vi "Date Start (XXXXXX).vi"(10 "13:00:00":string="00:00:00", 11 "Datetime":timestamp) -> (1 "檔名":string, 3 "Date + 00:00:00":timestamp)   [LabVIEW 2019]
panel:
  out "date string":string
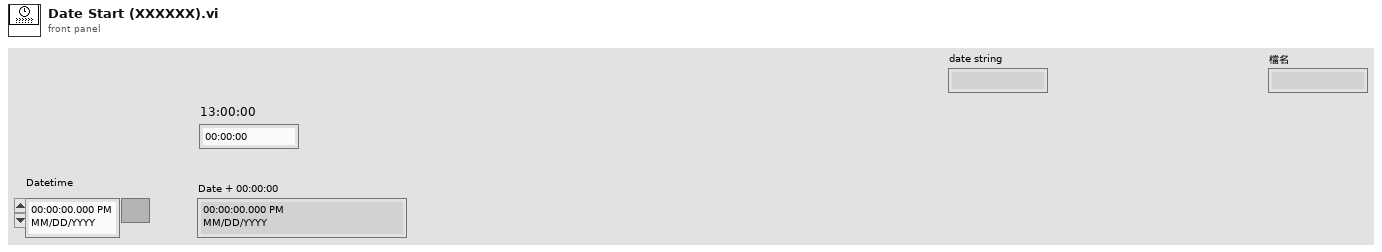
[diagram p1: front panel]
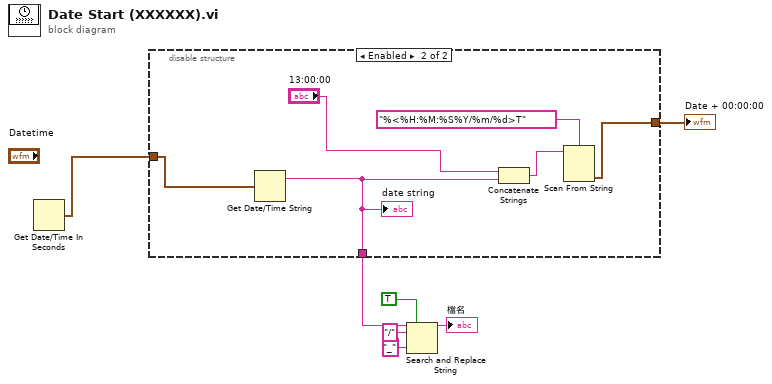
[diagram p0: block diagram]
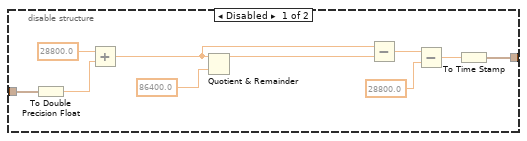
[diagram p2: hidden frame]
diagram:
  n1 = Get Date/Time In Seconds() -> (seconds since 1Jan1904=w1:timestamp)
  n2 = disable-structure shown="Enabled" {
    disable-tunnel: [w17 w20] -> w7
    disable-tunnel: w1 -> [w8 w21]
    disable-tunnel: [_ w19] -> w6
    frame Disabled {
      n3 = To Double Precision Float(number=w8) -> (double precision float=w11:dbl)
      n4 = Add(x=28800.0, y=w11) -> (x+y=w10:dbl)
      n5 = Quotient & Remainder(x=w10, y=86400.0) -> (x-y*floor(x/y)=w9:dbl)  [unwired: 1 out]
      n6 = Subtract(x=w10, y=w9) -> (x-y=w13:dbl)
      n7 = Subtract(x=w13, y=28800.0) -> (x-y=w14:dbl)
      n8 = To Time Stamp(1:w14) -> (0:w17:timestamp)
    }
    frame Enabled {
      n9 = Get Date/Time String(seconds (now)=w21) -> (date string=w19:string)  [unwired: 2 in, 1 out]
      "date string" <- w19
      n10 = Concatenate Strings("13:00:00", w19) -> (w23:string)
      n11 = Scan From String(format string="%<%H:%M:%S%Y/%m/%d>T", input string=w23) -> (output 1=w20:timestamp)  [unwired: 3 in, 3 out]
    }
  }
  "Date + 00:00:00" <- w7
  n12 = Search and Replace String(replace all?=TRUE ("replace all? (F)"), input string=w6, search string="/", replace string="_" ("replace string (\"\")")) -> (result string=→"檔名":string)  [unwired: 4 in, 3 out]
